vi "Get HDI Pad Local Coordinates.vi"(8 "error in":errorcluster, 9 "ROC Pad Number":i32, 10 "ROC":i32, 11 "Config Location":path) -> (0 "error out":errorcluster, 2 "Pad Local Coordinates":refnum<class "Vec3d Class.lvclass">)   [LabVIEW 2011]
uses:
  Vec3d Class/Vec3d Class.lvclass
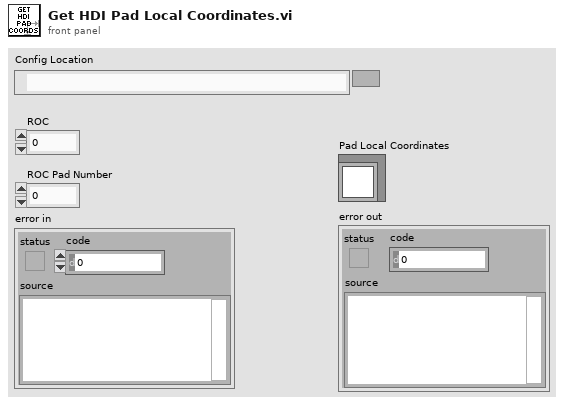
[diagram p1: front panel]
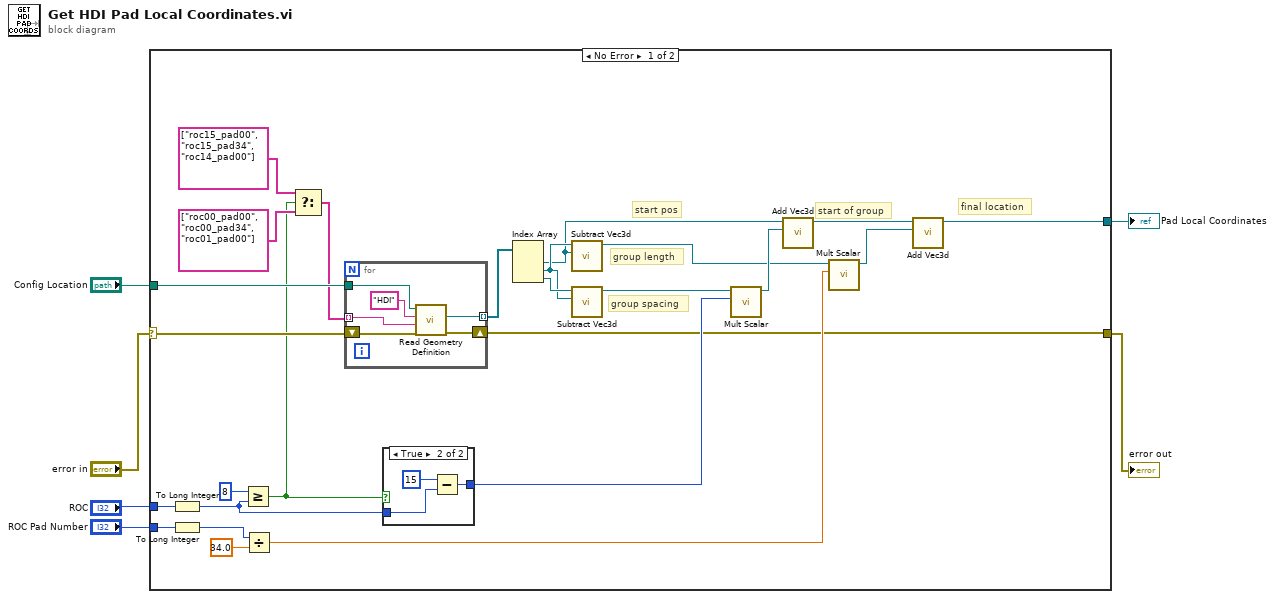
[diagram p0: block diagram]
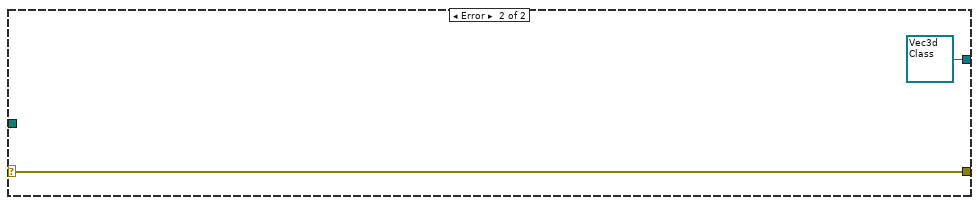
[diagram p3: hidden frame]
diagram:
  n1 = case shown="No Error" "error in" {
    selector: "error in" -> [w31 w43]
    tunnel: "Config Location" -> [w30 _]
    tunnel: "ROC" -> [w17 _]
    tunnel: "ROC Pad Number" -> [w15 _]
    tunnel: [w8 refnum<class "Vec3d Class.lvclass"> refnum ("Vec3d Class out")] -> w4
    tunnel: [w7 w43] -> w3
    frame No Error {
      # "final location"
      # "start of group"
      # "group spacing"
      # "group length"
      # "start pos"
      n2 = To Long Integer(number=w17) -> (32bit integer=w16:i32)
      n3 = To Long Integer(number=w15) -> (32bit integer=w13:i32)
      n4 = Greater Or Equal?(x=8, y=w16) -> (x >= y?=w20:bool)
      n5 = Divide(x=w13, y=34.0) -> (x/y=w10:dbl)
      n6 = Select(t=string[] ["roc15_pad00", "roc15_pad34", "roc14_pad00"], s=w20, f=string[] ["roc00_pad00", "roc00_pad34", "roc01_pad00"]) -> (s? t:f=w25:string[])
      n7 = for {
        tunnel: w30 -> [w41]
        shift-right: [w39] -> w7
        shift-left: w31 -> [w40]
        tunnel: w25 -> [w37] mode=indexing
        tunnel: [w36] -> w26 mode=indexing
        n8 = call "Read Geometry Definition.vi"("error in"=w40, "Feature"=w37, "Part"="HDI", "Config Location"=w41) -> ("error out"=w39:errorcluster, "Feature Coordinates"=w36:refnum<class "Vec3d Class.lvclass">)  [unwired: 6 in]
      }
      n9 = case shown="True" w20 {
        tunnel: w16 -> [w32 w35]
        tunnel: [w32 w33] -> w19
        frame False {
        }
        frame True {
          n10 = Subtract(x=15, y=w35) -> (x-y=w33:i32)
        }
      }
      n11 = Index Array(array=w26) -> (element #1=w22:refnum<class "Vec3d Class.lvclass">, element #2=w28:refnum<class "Vec3d Class.lvclass">, element #3=w29:refnum<class "Vec3d Class.lvclass">)  [unwired: 3 in]
      n12 = call "Subtract Vec3d.vi"("Vec3d in 2"=w22, "Vec3d in 1"=w28) -> ("Vec3d Class out"=w9:refnum<class "Vec3d Class.lvclass">)  [unwired: 8 in, 1 out]
      n13 = call "Subtract Vec3d.vi"("Vec3d in 2"=w28, "Vec3d in 1"=w29) -> ("Vec3d Class out"=w21:refnum<class "Vec3d Class.lvclass">)  [unwired: 8 in, 1 out]
      n14 = call-dynamic "Mult Scalar.vi"("Scale"=w19, "Vec3d in"=w21) -> ("Vec3d out"=w18:refnum<class "Vec3d Class.lvclass">)  [unwired: 8 in, 1 out]
      n15 = call-dynamic "Add Vec3d.vi"(10:"Vec3d Class in"=w18, 11:"Vec3d Class in"=w22) -> ("Vec3d Class out"=w11:refnum<class "Vec3d Class.lvclass">)  [unwired: 8 in, 1 out]
      n16 = call-dynamic "Mult Scalar.vi"("Scale"=w10, "Vec3d in"=w9) -> ("Vec3d out"=w12:refnum<class "Vec3d Class.lvclass">)  [unwired: 8 in, 1 out]
      n17 = call-dynamic "Add Vec3d.vi"(10:"Vec3d Class in"=w12, 11:"Vec3d Class in"=w11) -> ("Vec3d Class out"=w8:refnum<class "Vec3d Class.lvclass">)  [unwired: 8 in, 1 out]
    }
    frame Error {
    }
  }
  "Pad Local Coordinates" <- w4
  "error out" <- w3
